vi "Display Anything JSON.vi"(0 "Data":variant) -> ()   [LabVIEW 2021]
uses:
  <vilib>/addons/_JKI.lib/Serialization/JSON/JKI JSON Serialization.lvlib
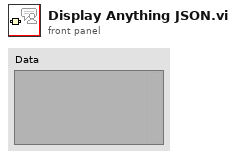
[diagram p1: front panel]
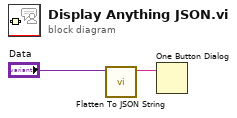
[diagram p0: block diagram]
diagram:
  n1 = call <vilib>:"Flatten To JSON String.vi"("Variant"="Data") -> ("JSON String"=w2:string)  [unwired: 9 in, 1 out]
  n2 = One Button Dialog(message=w2) -> ()  [unwired: 1 in, 1 out]
